vi "smart decimate  - V2.vi"(7 "number of 2D grid points":i32=300, 8 "complex region":T1={"max re"=0.984067684418521, "min re"=-2.0159323155814786, "max im"=3.076570113964653, "min im"=0.06786753047429528, "delta re"=2.9999999999999996, "delta im"=3.008702583490358, "center re"=-0.5159323155814788, "delta  z"=1.5722188222194742+0.0i, "center im"=0.0, "center z"=0.0+0.0i, "d im"=0.0, "d re"=0.0, "d z"=0.0+0.0i}, 9 "omega in":dbl[](array[numeric]), 10 "decimation threshold":i32=3, 11 "z in":cdb[](array[numeric])) -> (0 "number of decimated elements":i32, 1 "decimated omega":dbl[](array[numeric]), 3 "decimated z":cdb[](array[numeric]))   [LabVIEW 2021]
uses:
  complex region.ctl
panel:
  in  "x + iy":cdb[](array[numeric])
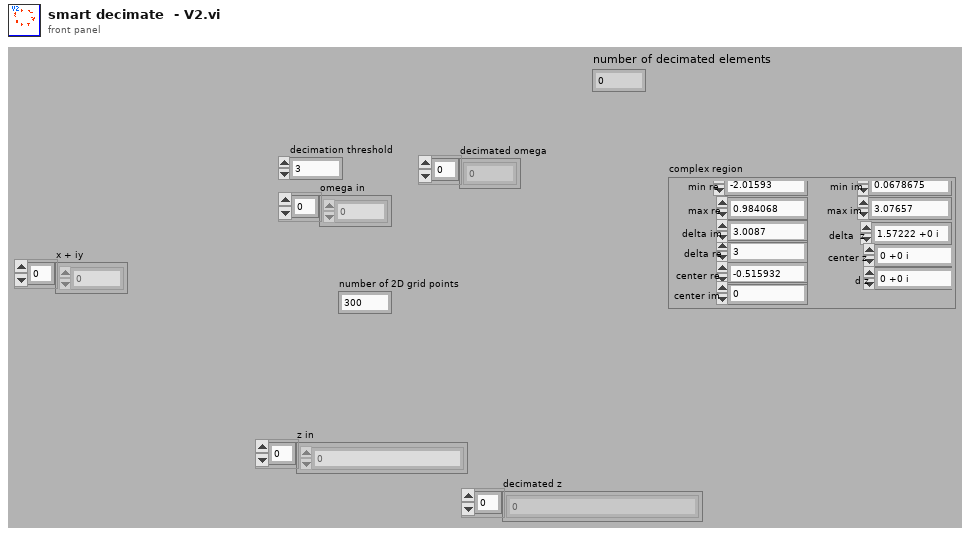
[diagram p1: front panel]
types:
  T1 = typedef "complex region.ctl" = cluster{"max re":dbl, "min re":dbl, "max im":dbl, "min im":dbl, "delta re":dbl, "delta im":dbl, "center re":dbl, "delta  z":cdb, "center im":dbl, "center z":cdb, "d im":dbl, "d re":dbl, "d z":cdb}
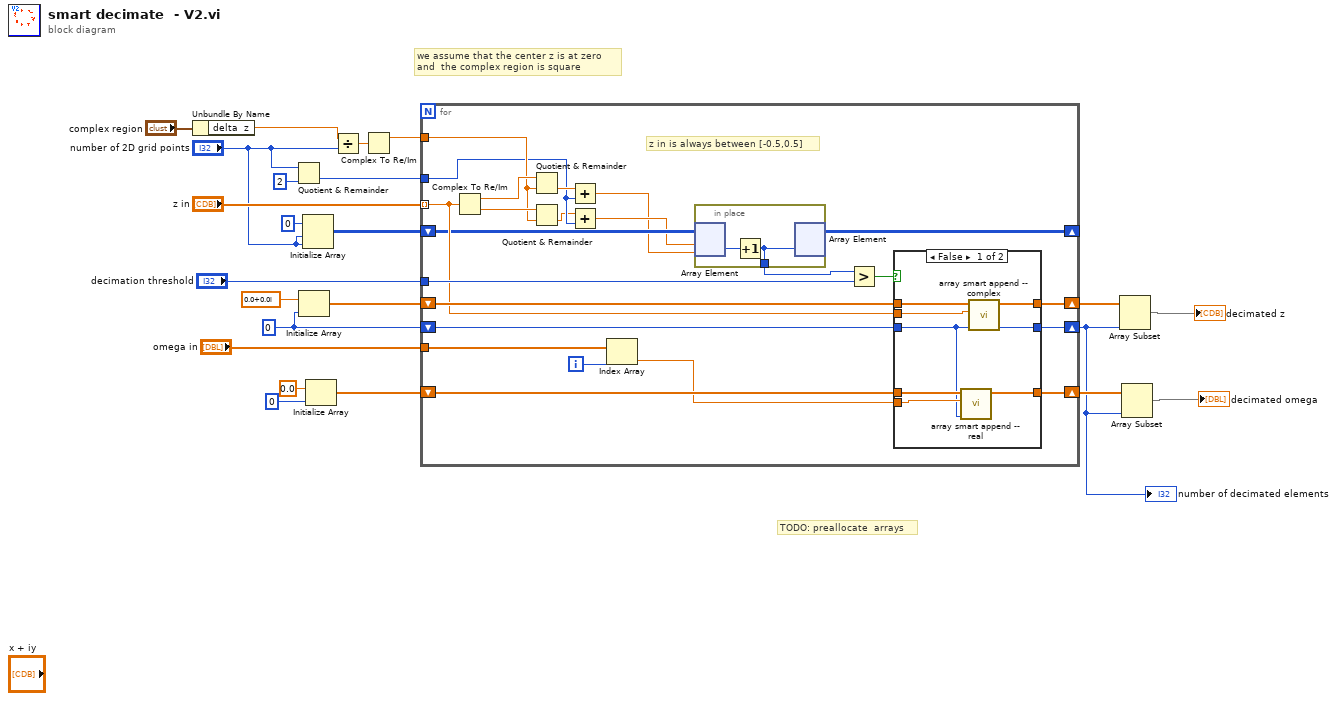
[diagram p0: block diagram]
diagram:
  w6 = 0 ("element")
  # "TODO: preallocate  arrays"
  # "we assume that the center z is at zero \nand  the complex region is square"
  n1 = Unbundle By Name("complex region") -> ("delta  z"=w12:cdb)
  n2 = Quotient & Remainder(x="number of 2D grid points", y=2) -> (floor(x/y)=w8:i32)  [unwired: 1 out]
  n3 = Initialize Array(cdb 0.0+0.0i ("element"), w6) -> (w21:cdb[])
  n4 = Initialize Array(i16 0 ("element"), "number of 2D grid points", "number of 2D grid points") -> (w20:i16[][])
  n5 = Initialize Array(0.0 ("element"), 0 ("element")) -> (w15:dbl[])
  n6 = Divide(x=w12, y="number of 2D grid points") -> (x/y=w13:cdb)
  n7 = Complex To Re/Im(x + iy=w13) -> (x=w11:dbl)  [unwired: 1 out]
  n8 = for {
    shift-right: [w45] -> w5
    shift-left: w21 -> [w44]
    tunnel: "z in" -> [w34] mode=indexing
    shift-right: [w25] -> _
    shift-left: w20 -> [w28]
    tunnel: "decimation threshold" -> [w43]
    tunnel: "omega in" -> [w42]
    shift-right: [w39] -> w3
    shift-left: w15 -> [w40]
    tunnel: w11 -> [w35]
    tunnel: w8 -> [w32]
    shift-right: [w29] -> w1
    shift-left: w6 -> [w30]
    i -> [w41]
    # "z in is always between [-0.5,0.5]"
    n9 = Complex To Re/Im(x + iy=w34) -> (x=w37:dbl, y=w36:dbl)
    n10 = Quotient & Remainder(x=w37, y=w35) -> (floor(x/y)=w33:dbl)  [unwired: 1 out]
    n11 = Quotient & Remainder(x=w36, y=w35) -> (floor(x/y)=w31:dbl)  [unwired: 1 out]
    n12 = Add(x=w33, y=w32) -> (x+y=w26:dbl)
    n13 = Add(x=w31, y=w32) -> (x+y=w27:dbl)
    n14 = Index Array(array=w42, index=w41) -> (element=w38:dbl)
    n15 = in-place {
      in-place-border: [w47] -> w24
      n16 = in-place-array #1(w28, w27, w26) -> (w48:i16)
      n17 = Increment(x=w48) -> (x+1=w47:i16)
      n18 = in-place-array #1(w47) -> (w25:i16[][])  [unwired: 2 out]
    }
    n19 = Greater?(x=w24, y=w43) -> (0:w46:bool)
    n20 = case shown="False" w46 {
      tunnel: [w55 w59] -> w45
      tunnel: w44 -> [w56 w59]
      tunnel: w34 -> [w54 _]
      tunnel: w40 -> [w52 w58]
      tunnel: [w50 w58] -> w39
      tunnel: w38 -> [w51 _]
      tunnel: w30 -> [w49 w57]
      tunnel: [w53 w57] -> w29
      frame False {
        n21 = call "array smart append -- real.vi"("last index"=w49, "Numeric"=w51, "Array"=w52) -> ("output array"=w50:dbl[])  [unwired: 7 in, 1 out]
        n22 = call "array smart append -- complex.vi"("last index"=w49, "Numeric"=w54, "Array"=w56) -> ("last index out"=w53:i32, "output array"=w55:cdb[])  [unwired: 7 in]
      }
      frame True {
      }
    }
  }
  "number of decimated elements" <- w1
  n23 = Array Subset(array=w5, length=w1) -> (→"decimated z":cdb[])  [unwired: 1 in]
  n24 = Array Subset(array=w3, length=w1) -> (→"decimated omega":dbl[])  [unwired: 1 in]
